vi "4431 - Read AND Write.vi"(4 "Reset":bool, 6 "AO Array":waveform(dbl)[](array[waveform]), 8 "error in (no error)":errorcluster, 9 "sampling info":cluster{"Fs":dbl, "#s":dbl}={"Fs"=1000.0, "#s"=1000.0} {"Fs" format="%.2p"}, 10 "AO Task":refnum<k21>[](array[refnum]), 11 "AI task":refnum<k21>[](array[refnum])=["", ""]) -> (0 "error out":errorcluster, 3 "Input Signals":waveform(dbl)[](array[waveform]))   [LabVIEW 2016]
uses:
  <vilib>/DAQmx/write.llb/DAQmx Write (Analog 1D Wfm NChan NSamp).vi
  <vilib>/DAQmx/read.llb/DAQmx Read (Analog 1D Wfm NChan NSamp).vi
  <vilib>/DAQmx/miscellaneous.llb/DAQmx Fill In Error Info.vi
  <resource>/objmgr/daqmx.rc
panel:
  out "AvailSampPerChan":u32[](array[numeric])
  out "AvailSampPerChan 4":u32
  out "AvailSampPerChan 3":u32
  out "AvailSampPerChan 2":u32
  out "AvailSampPerChan 1":u32
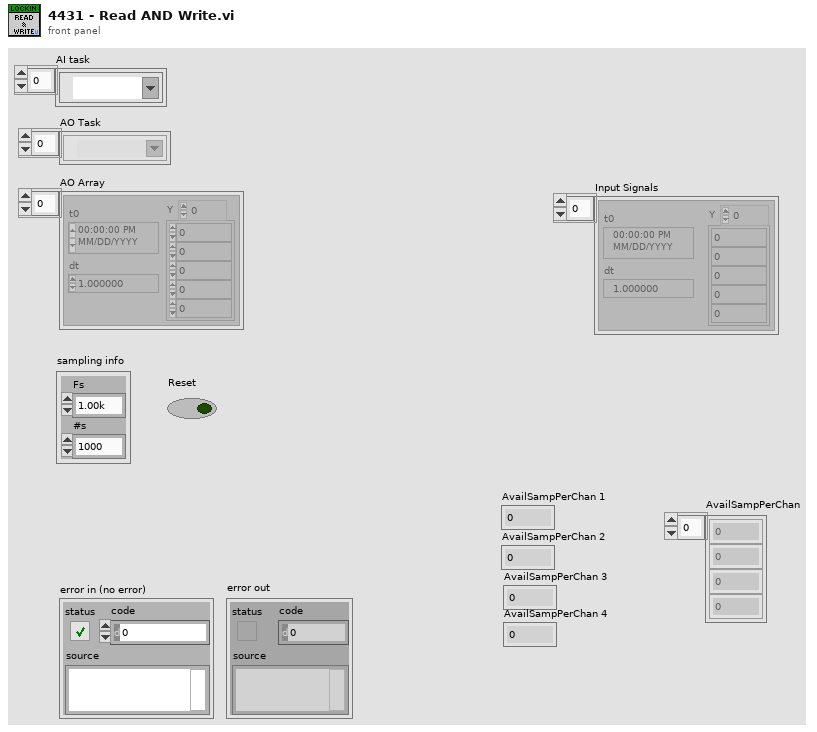
[diagram p1: front panel]
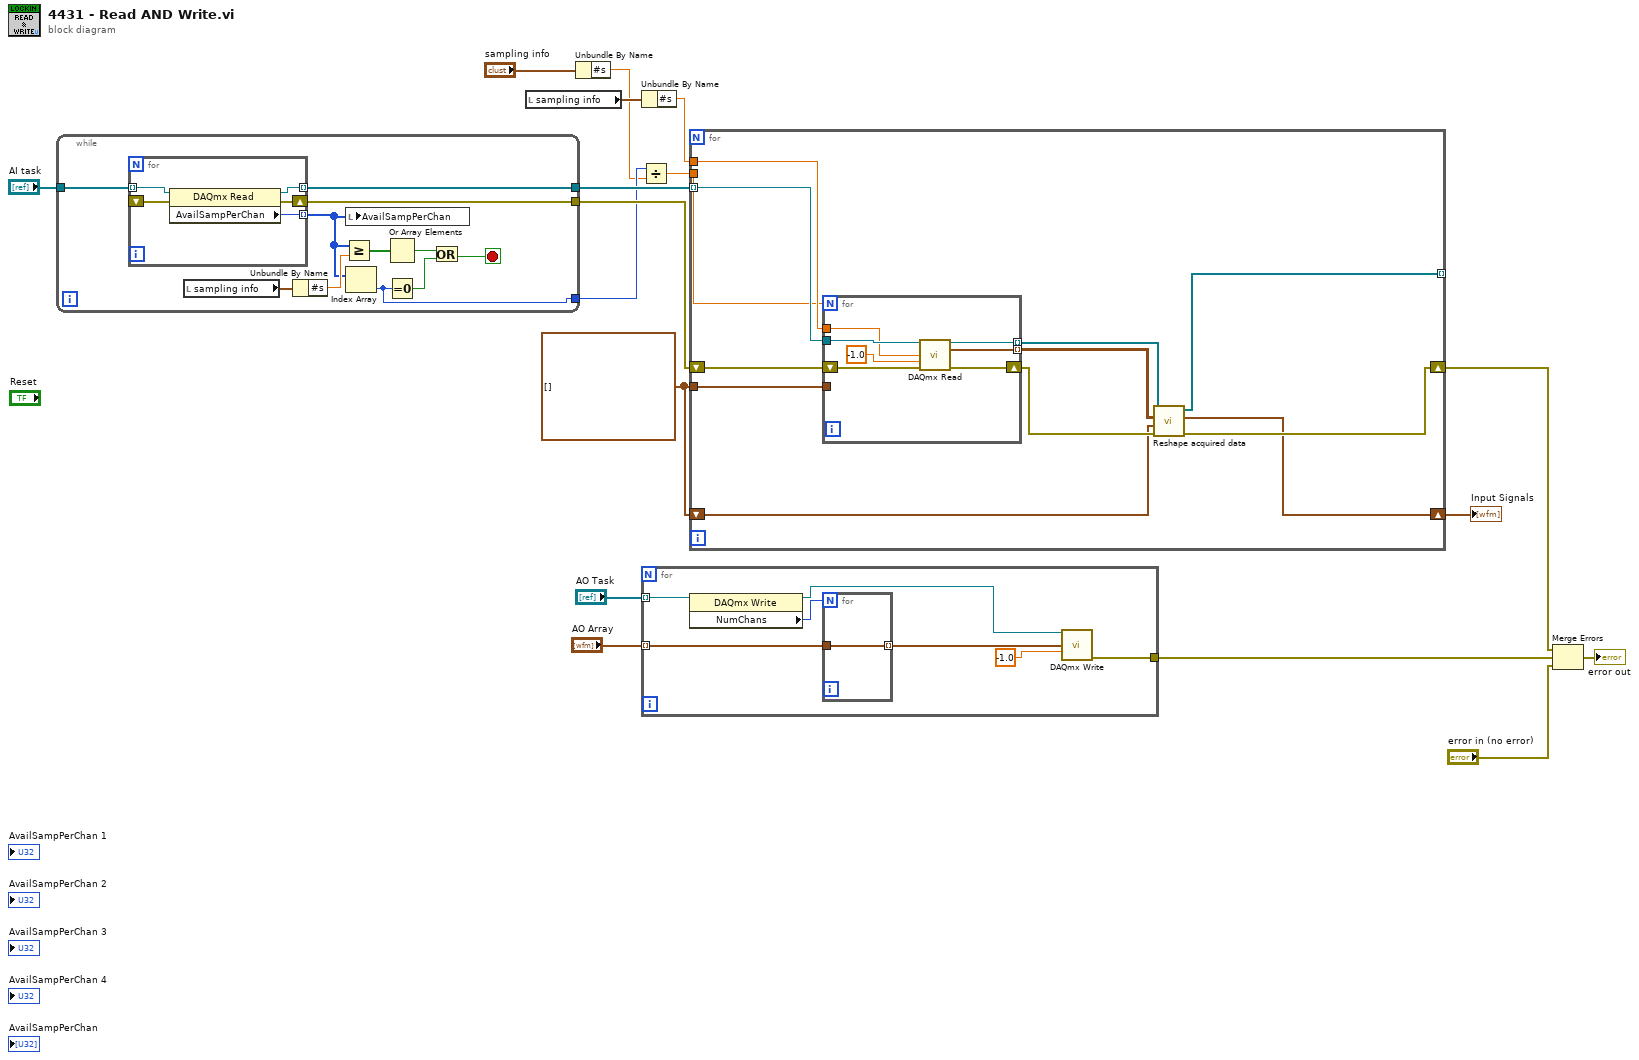
[diagram p0: block diagram]
diagram:
  w2 = waveform(dbl)[] []
  n1 = while {
    tunnel: "AI task" -> [w25]
    tunnel: [w24] -> w14
    tunnel: [w23] -> w12
    tunnel: [w18] -> w9
    stop <- w19 stop-if-true
    n2 = for {
      tunnel: [w33] -> w22 mode=indexing
      shift-right: [w31] -> w23
      shift-left: _ -> [w32]
      tunnel: w25 -> [w30] mode=indexing
      tunnel: [w29] -> w24 mode=indexing
      n3 = property class="DAQmx Read"(reference=w30, error in=w32) -> (reference out=w29:refnum<k21>, error out=w31:errorcluster, "AvailSampPerChan"=w33:u32)
    }
    n4 = local read "sampling info"() -> (w28:cluster{"Fs":dbl, "#s":dbl})
    n5 = Unbundle By Name(w28) -> ("#s"=w27:dbl)
    n6 = Greater Or Equal?(x=w22, y=w27) -> (x >= y?=w26:bool[])
    n7 = local write "AvailSampPerChan"(w22) -> ()
    n8 = Index Array(array=w22) -> (element=w18:u32)  [unwired: 1 in]
    n9 = Or Array Elements(Boolean array=w26) -> (logical OR=w20:bool)
    n10 = Equal To 0?(x=w18) -> (x = 0?=w21:bool)
    n11 = Or(x=w20, y=w21) -> (x .or. y?=w19:bool)
  }
  n12 = local read "sampling info"() -> (w13:cluster{"Fs":dbl, "#s":dbl})
  n13 = Unbundle By Name("sampling info") -> ("#s"=w8:dbl)
  n14 = Divide(x=w9, y=w8) -> (x/y=w7:dbl)
  n15 = Unbundle By Name(w13) -> ("#s"=w10:dbl)
  n16 = for {
    tunnel: "AO Array" -> [w38] mode=indexing
    tunnel: "AO Task" -> [w40] mode=indexing
    tunnel: [w34] -> w4
    n17 = property class="DAQmx Write"(reference=w40) -> (reference out=w35:refnum<k21>, "NumChans"=w39:u32)  [unwired: 1 in, 1 out]
    n18 = for {
      N: w39 -> [_]
      tunnel: w38 -> [w41]
      tunnel: [w41] -> w36 mode=indexing
    }
    n19 = call-poly <vilib>:"DAQmx Write.vi"("task/channels in"=w35, "data"=w36, "timeout"=-1.0) -> ("error out"=w34:errorcluster)  [unwired: 10 in, 2 out]
  }
  n20 = for {
    tunnel: w14 -> [w53] mode=indexing
    tunnel: w10 -> [w51]
    tunnel: w7 -> [w50]
    shift-right: [w46] -> w11
    shift-left: w12 -> [w52]
    tunnel: w2 -> [w49]
    shift-right: [w44] -> w1
    shift-left: w2 -> [w43]
    tunnel: [w45] -> _ mode=indexing
    n21 = for {
      N: w50 -> [_]
      shift-right: [w58] -> w48
      shift-left: w52 -> [w59]
      tunnel: w53 -> [w57]
      tunnel: [w56] -> w47 mode=indexing
      tunnel: w51 -> [w55]
      tunnel: w49 -> [_]
      tunnel: [w54] -> w42 mode=indexing
      n22 = call-poly <vilib>:"DAQmx Read.vi"("task/channels in"=w57, "number of samples per channel"=w55, "timeout"=-1.0, "error in"=w59) -> ("task out"=w56:refnum<k21>, "data"=w54:waveform(dbl)[], "error out"=w58:errorcluster)  [unwired: 9 in]
    }
    n23 = call "Reshape acquired data.vi"("error in (no error)"=w48, "Array in"=w43, "data"=w42, "Array 4"=w47) -> ("error out"=w46:errorcluster, "Array out"=w44:waveform(dbl)[], "Array 3"=w45:refnum<k21>[])  [unwired: 5 in]
  }
  "Input Signals" <- w1
  n24 = Merge Errors(w11, w4, "error in (no error)") -> (→"error out":errorcluster)
